vi "SaveWWWImages2.vi"(7 "Tab charts":refnum<vi>, 9 "Image Data 2":T1, 10 "Destination":path, 11 "VI in":refnum<vi>) -> ()   [LabVIEW 2017]
uses:
  Web Imge control.ctl
panel:
  out "Write Imegtime":u32
  out "get Imegtime":u32
  out "Time":u32
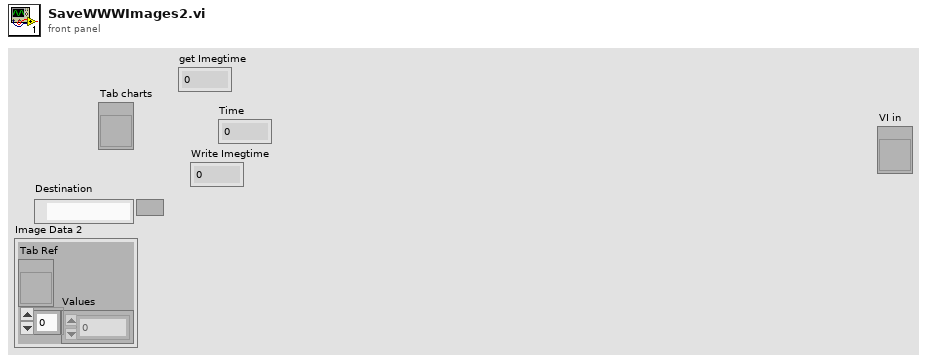
[diagram p1: front panel]
types:
  T1 = typedef "Web Imge control.ctl" = cluster{"Tab Ref":refnum<vi>, "Values":i32[]}
  T2 = typedef "imagedata.ctl" = cluster{"image type":i32, "image depth":i32, "image":u8[], "mask":u8[], "colors":u32[], "Rectangle":cluster{"left":i16, "top":i16, "right":i16, "bottom":i16}}
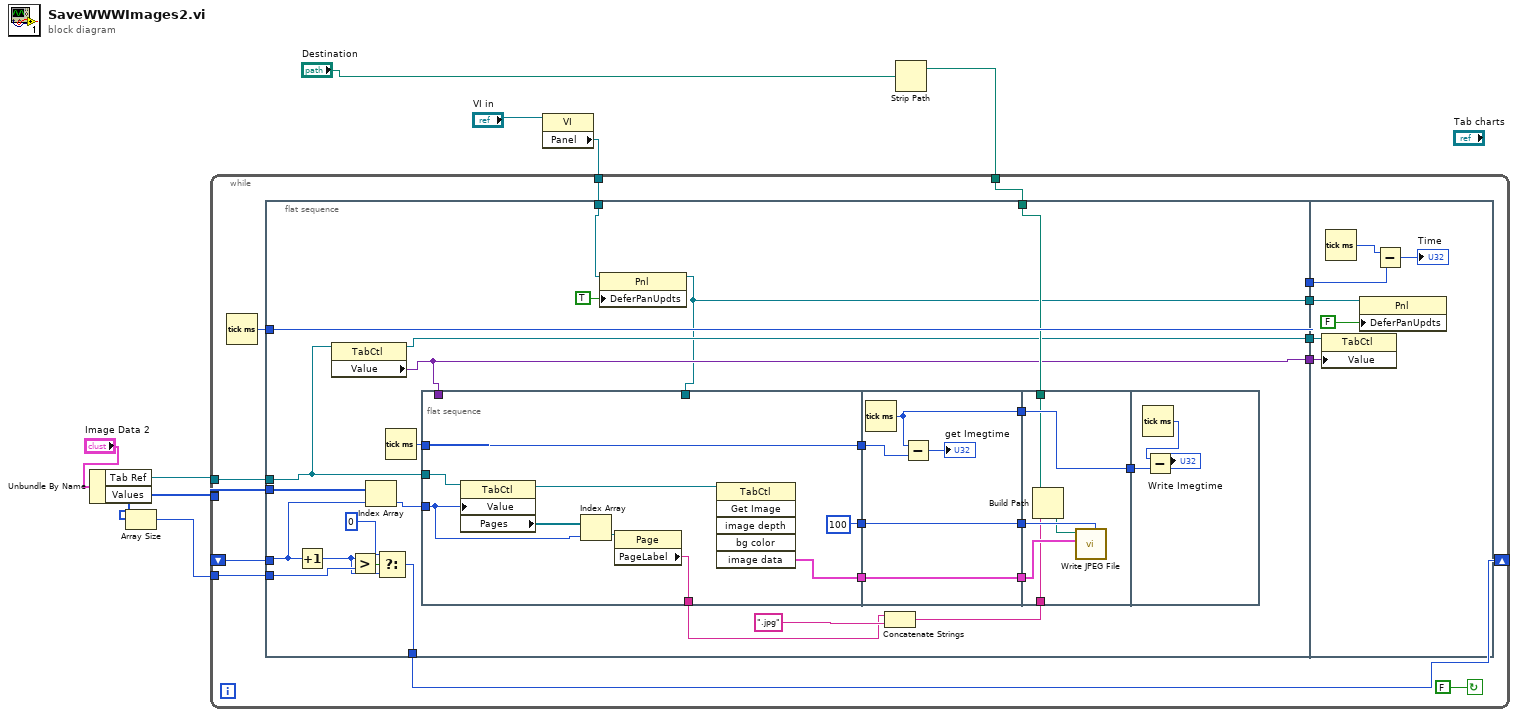
[diagram p0: block diagram]
diagram:
  n1 = Unbundle By Name("Image Data 2") -> ("Tab Ref"=w4:refnum<vi>, "Values"=w2:i32[])
  n2 = Array Size(array=w2) -> (size(s)=w1:i32)
  n3 = property class="VI"(reference="VI in") -> ("Panel"=w5:refnum<vi>)  [unwired: 1 in, 2 out]
  n4 = Strip Path(path="Destination") -> (stripped path=w6:path)  [unwired: 1 out]
  n5 = while {
    tunnel: w6 -> [w18]
    tunnel: w5 -> [w17]
    shift-right: [w9] -> _
    shift-left: _ -> [w11]
    tunnel: w2 -> [w12]
    tunnel: w4 -> [w13]
    tunnel: [w12] -> _
    tunnel: w1 -> [w10]
    stop <- FALSE continue-if-true
    n6 = Tick Count (ms)() -> (millisecond timer value=w20:u32)
    n7 = flat-sequence {
      tunnel: [w48] -> w21
      tunnel: w20 -> [w48]
      tunnel: w18 -> [w47]
      tunnel: w17 -> [w45]
      tunnel: [w22] -> w16
      tunnel: [w44] -> w15
      tunnel: [w29] -> w14
      tunnel: w13 -> [w31]
      tunnel: w12 -> [w30]
      tunnel: w11 -> [w24]
      tunnel: w10 -> [w27]
      tunnel: [w25] -> w9
      tunnel: w21 -> [w77]
      tunnel: w16 -> [w74]
      tunnel: w15 -> [w73]
      tunnel: w14 -> [w72]
      frame #0 {
        n8 = Increment(x=w24) -> (x+1=w23:i32)
        n9 = property class="TabCtl"(reference=w31) -> (reference out=w44:refnum<vi>, "Value"=w29:variant)  [unwired: 1 in, 1 out]
        n10 = Greater?(x=w23, y=w27) -> (0:w28:bool)
        n11 = Index Array(array=w30, index=w24) -> (element=w32:i32)
        n12 = Select(t=0, s=w28, f=w23) -> (s? t:f=w25:i32)
        n13 = Tick Count (ms)() -> (millisecond timer value=w35:u32)
        n14 = flat-sequence {
          tunnel: [w56] -> w43
          tunnel: [100 ("quality (80)")] -> w42
          tunnel: [w54] -> w41
          tunnel: w35 -> [w54]
          tunnel: w32 -> [w53]
          tunnel: [w50] -> w34
          tunnel: w31 -> [w49]
          tunnel: w29 -> [_]
          tunnel: w22 -> [_]
          tunnel: w43 -> [w62]
          tunnel: [w62] -> w40
          tunnel: w42 -> [w61]
          tunnel: [w61] -> w39
          tunnel: w41 -> [w60]
          tunnel: [w58] -> w38
          tunnel: w40 -> [w67]
          tunnel: w39 -> [w68]
          tunnel: w38 -> [w66]
          tunnel: [w66] -> w37
          tunnel: w47 -> [w65]
          tunnel: w33 -> [w63]
          tunnel: w37 -> [w69]
          frame #0 {
            n15 = property class="TabCtl"(reference=w49, "Value"=w53) -> (reference out=w57:refnum<vi>, "Pages"=w52:refnum<vi>[])  [unwired: 1 in, 1 out]
            n16 = Index Array(array=w52, index=w53) -> (element=w51:refnum<vi>)
            n17 = property class="Page"(reference=w51) -> ("PageLabel"=w50:string)  [unwired: 1 in, 2 out]
            n18 = invoke class="TabCtl" method="Get Image"(reference=w57) -> ("image data"=w56:T2)  [unwired: 5 in, 5 out]
          }
          frame #1 {
            n19 = Tick Count (ms)() -> (millisecond timer value=w58:u32)
            n20 = Subtract(x=w58, y=w60) -> (x-y=→"get Imegtime":u32)
          }
          frame #2 {
            n21 = Build Path(base path=w65, name or relative path=w63) -> (appended path=w64:path)
            n22 = call <vilib>:"Write JPEG File.vi"("quality (80)"=w68, "image data"=w67, "path to JPEG file"=w64) -> ()  [unwired: 7 in, 2 out]
          }
          frame #3 {
            n23 = Tick Count (ms)() -> (millisecond timer value=w70:u32)
            n24 = Subtract(x=w70, y=w69) -> (x-y=→"Write Imegtime":u32)
          }
        }
        n25 = property class="Pnl"(reference=w45, "DeferPanUpdts"=TRUE ("Defer Panel Updates")) -> (reference out=w22:refnum<vi>)  [unwired: 1 in, 1 out]
        n26 = Concatenate Strings(w34, ".jpg" ("string")) -> (w33:string)
      }
      frame #1 {
        n27 = property class="TabCtl"(reference=w73, "Value"=w72) -> ()  [unwired: 1 in, 2 out]
        n28 = Tick Count (ms)() -> (millisecond timer value=w78:u32)
        n29 = property class="Pnl"(reference=w74, "DeferPanUpdts"=FALSE ("Defer Panel Updates")) -> ()  [unwired: 1 in, 2 out]
        n30 = Subtract(x=w78, y=w77) -> (x-y=→"Time":u32)
      }
    }
  }
